vi "Get Counter.vi"() -> ()   [LabVIEW 2018]
uses:
  <instrlib>/AltonTech MALT/Public/Types/MALT Family Codes.ctl
  <instrlib>/AltonTech MALT/AltonTech MALT200817.lvlib
panel:
  out "PortCounters":u32[](array[numeric])
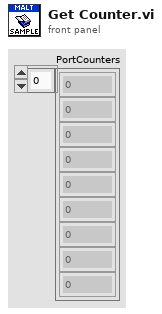
[diagram p1: front panel]
types:
  T1 = typedef "AltonTech MALT200817.lvlib/MALT Family Codes.ctl" = enum32{"-", "YAV90832", "YAV904X8", "MALT132", "YAV91616", "MALT16PIN", "YAV90096", "YAV90HVT", "YAV90CLR", "YAV90128", "YAV90PNE", "YAVCANCON", "YAV91775", "YAV90XXX", "YAV90MMU", "H730050", "H710060", "H710061", "YAV90304", "MMI", "YAV90060", "MALT160T", "YAV90059", "Not Defined"}
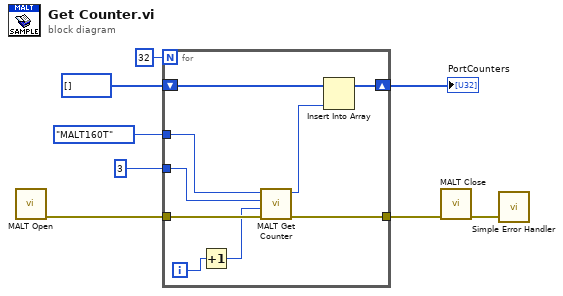
[diagram p0: block diagram]
diagram:
  n1 = call <instrlib>:"MALT Open.vi"() -> ("error out"=w7:errorcluster)  [unwired: 11 in]
  n2 = for {
    N: 32 -> [_]
    tunnel: w7 -> [w17]
    tunnel: [w16] -> w6
    tunnel: MALT_Family_Codes."MALT160T" ("FamilyCode") -> [w15]
    tunnel: 3 ("Address") -> [w14]
    shift-right: [w9] -> w2
    shift-left: u32[] [] -> [w11]
    i -> [w13]
    n3 = Increment(x=w13) -> (x+1=w12:i32)
    n4 = call <instrlib>:"MALT Get Counter.vi"("error in"=w17, "Port"=w12, "Address"=w14, "FamilyCode"=w15) -> ("error out"=w16:errorcluster, "Value"=w10:u32)  [unwired: 6 in]
    n5 = Insert Into Array(array=w11, new element=w10) -> (w9:u32[])  [unwired: 1 in]
  }
  "PortCounters" <- w2
  n6 = call <instrlib>:"MALT Close.vi"("error in"=w6) -> ("error out"=w8:errorcluster)  [unwired: 10 in]
  n7 = call <vilib>:"Simple Error Handler.vi"("error in (no error)"=w8) -> ()  [unwired: 4 in, 5 out]
